vi "Config SPI Digital Lines.vi"(8 "error in":errorcluster, 11 "SPI DIO Lines":T1={"SCLK"="Port0/DIO0", "MISO"="Port0/DIO1", "MOSI"="Port0/DIO2", "CS 0"="Port0/DIO4", "CS 1"="Port0/DIO5", "CS 2"="Port0/DIO6", "CS 3"="Port0/DIO7", "CS 4"="Port0/DIO8", "CS 5"="Port0/DIO9"}) -> (0 "error out":errorcluster, 3 "Chip Select DIO Lines":T1={"SCLK"="Port0/DIO3", "MISO"="Port0/DIO3", "MOSI"="Port0/DIO3", "CS 0"="Port0/DIO4", "CS 1"="Port0/DIO4", "CS 2"="Port0/DIO1", "CS 3"="Port0/DIO4", "CS 4"="Port0/DIO4", "CS 5"="Port0/DIO4"})   [LabVIEW 2014]
uses:
  <vilib>/SPIAPI/DIO/SPI Digital IO Lines.ctl
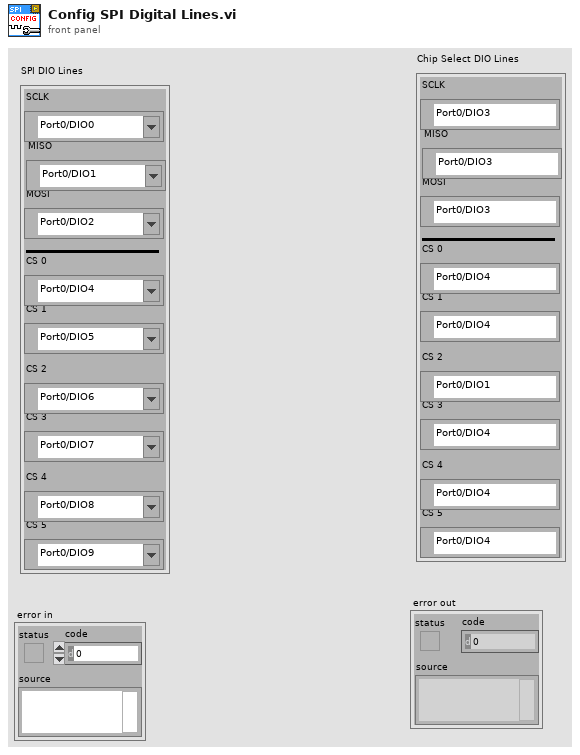
[diagram p1: front panel]
types:
  T1 = typedef "SPI Digital IO Lines.ctl" = cluster{"SCLK":refnum<k21>, "MISO":refnum<k21>, "MOSI":refnum<k21>, "CS 0":refnum<k21>, "CS 1":refnum<k21>, "CS 2":refnum<k21>, "CS 3":refnum<k21>, "CS 4":refnum<k21>, "CS 5":refnum<k21>}
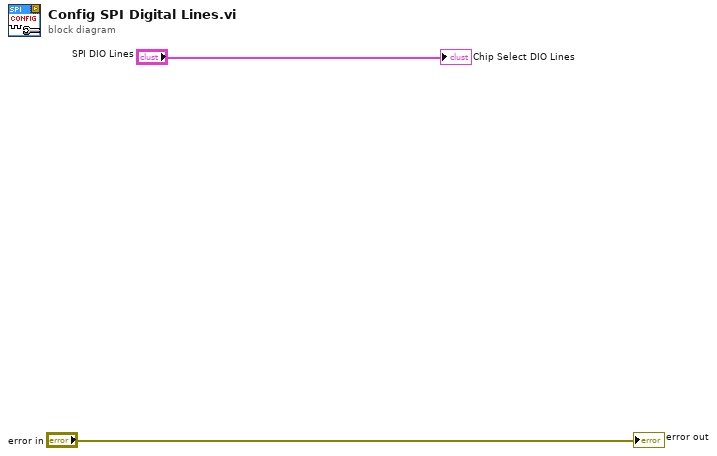
[diagram p0: block diagram]
diagram:
  "Chip Select DIO Lines" <- "SPI DIO Lines"
  "error out" <- "error in"
